vi "Stepper Mover.vi"() -> ()   [LabVIEW 2020]
doc: "Use this template to build a producer/consumer design pattern with events to produce queue items. Use this design pattern instead of the User Interface Event Handler pattern for user interfaces when you want to execute code asynchronously in response to an event without slowing the user interface responsiveness."
panel:
  out "Timeout error":bool
  out "error out":errorcluster
  in  "Velocity":i32
  in  "Init":bool
  in  "Set to Zero":bool
  in  "Stop Motor":bool
  out "Moving":bool
  out "Current Top Position":dbl format="%.1f"
  out "Current Bottom Position":dbl format="%.4f"
  in  "Instrument Address":refnum<visa-resource-name>
  in  "Rotator":T1(ring)=enum."System B 50 mm Magnet"
  in  "Move to Bottom Position (deg or in)":dbl format="%.4f"
  in  "Move to  Top Position (deg)":dbl format="%.1f"
  in  "stop":bool
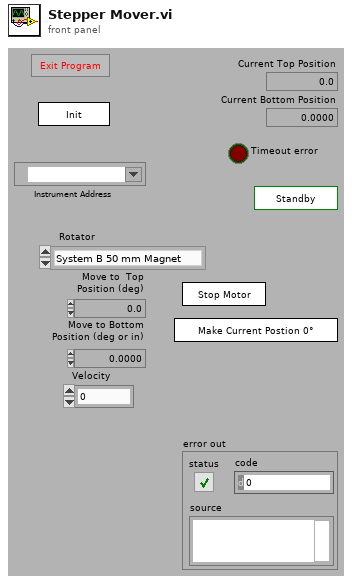
[diagram p1: front panel]
types:
  T1 = enum16{"Dilution Fridge SCM 1", "System A SCM 2", "System B 50 mm Magnet", "He-3 32 mm Magnet", "Portable Dil Fridge Rotator", "Linear Position", "System E Probe 1"}
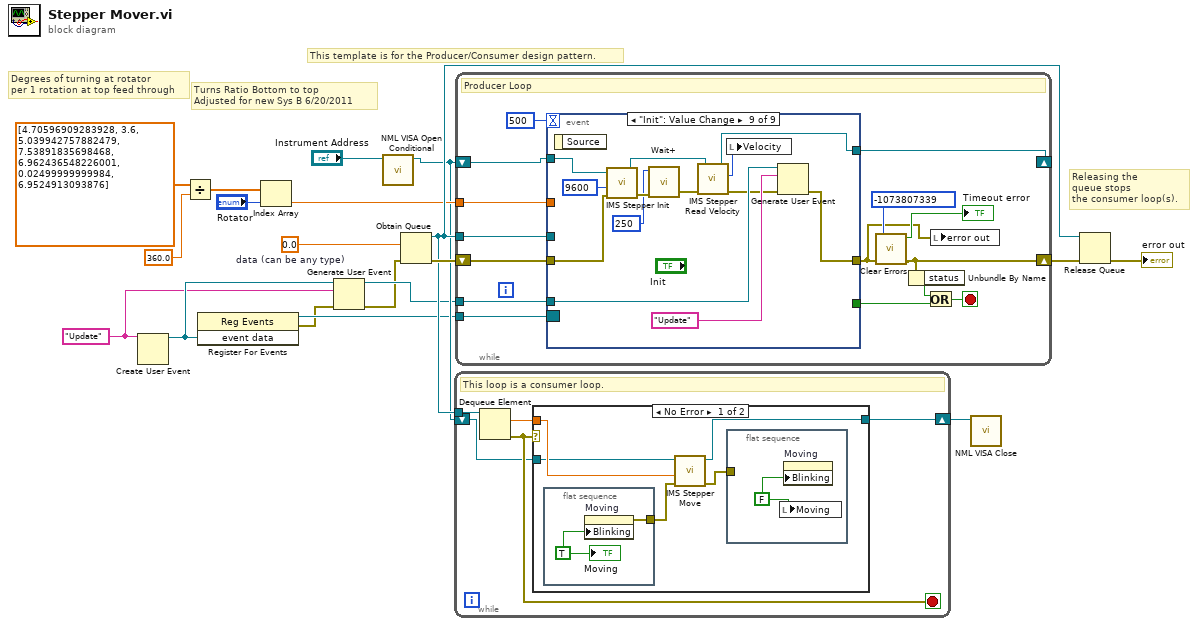
[diagram p0: block diagram]
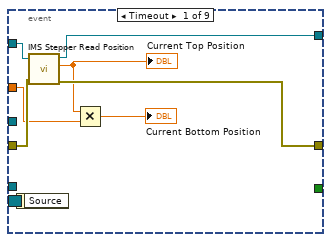
[diagram p3: hidden frame]
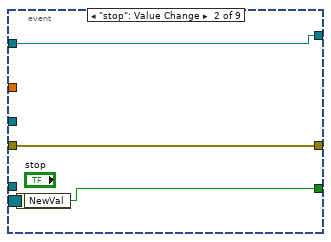
[diagram p4: hidden frame]
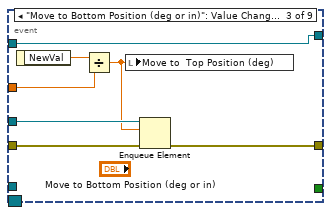
[diagram p5: hidden frame]
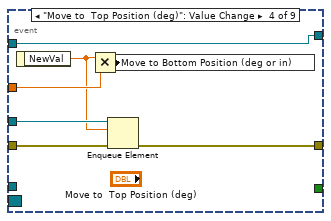
[diagram p6: hidden frame]
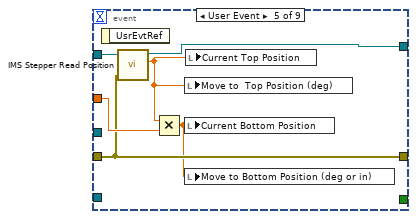
[diagram p7: hidden frame]
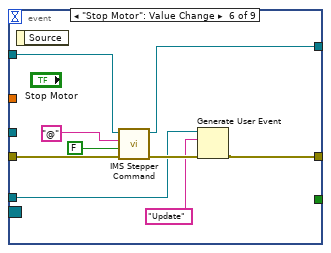
[diagram p8: hidden frame]
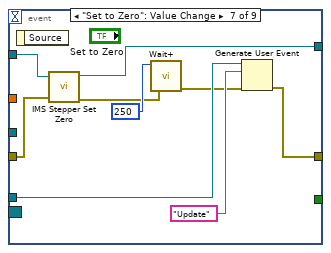
[diagram p9: hidden frame]
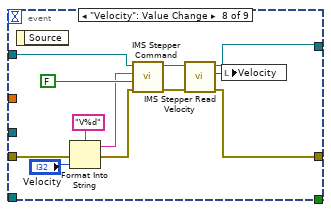
[diagram p10: hidden frame]
diagram:
  w6 = "Update" ("event data")
  w17 = 0.0  # data (can be any type)
  # "Degrees of turning at rotator\nper 1 rotation at top feed through"
  # "Turns Ratio Bottom to top\nAdjusted for new Sys B 6/20/2011"
  # "Releasing the\nqueue stops\nthe consumer loop(s)."
  # "This template is for the Producer/Consumer design pattern."
  n1 = Create User Event(user event datatype=w6) -> (user event=w9:refnum<user-event>)  [unwired: 1 in, 1 out]
  n2 = Divide(x=dbl[] [4.70596909283928, 3.6, 5.039942757882479, 7.53891835698468, 6.962436548226001, 0.02499999999984, 6.9524913093876] ("array"), y=360.0) -> (x/y=w2:dbl[])
  n3 = register-events(w9) -> (reference out=w11:refnum<event-registration>, error out=w10:errorcluster)  [unwired: 2 in]
  n4 = Index Array(array=w2, index="Rotator") -> (element=w13:dbl)
  n5 = Generate User Event(user event=w9, event data cluster=w6, error in=w10) -> (user event out=w8:refnum<user-event>, error out=w7:errorcluster)  [unwired: 1 in]
  n6 = call "NML VISA Open Conditional.vi"("VISA resource name"="Instrument Address") -> ("dup VISA Session"=w12:refnum<visa-resource-name>)  [unwired: 8 in, 2 out]
  n7 = Obtain Queue(element data type=w17, error in (no error)=w7) -> (queue out=w16:refnum<queue>, error out=w19:errorcluster)  [unwired: 3 in, 1 out]
  n8 = while {
    tunnel: w16 -> [w24]
    shift-right: [w20] -> w1
    shift-left: w12 -> [w21]
    stop <- w23 stop-if-true
    # "This loop is a consumer loop."
    n9 = Dequeue Element(queue=w24) -> (element=w22:dbl, error out=w23:errorcluster)  [unwired: 2 in, 2 out]
    n10 = case shown="No Error" w23 {
      tunnel: w22 -> [w29 _]
      tunnel: w21 -> [w28 w33]
      tunnel: [w25 w33] -> w20
      frame No Error {
        n11 = flat-sequence {
          tunnel: [w30] -> w27
          frame #0 {
            w31 = TRUE ("Moving")
            n12 = property on="Moving" class="Bool (strict)"("Blinking"=w31) -> (error out=w30:errorcluster)  [unwired: 2 in, 1 out]
            "Moving" <- w31
          }
        }
        n13 = call "IMS Stepper Move.vi"("error in (no error)"=w27, "Distance"=w29, "Instrument Address"=w28) -> ("error out"=w26:errorcluster, "Instrument Address Out"=w25:refnum<visa-resource-name>)  [unwired: 4 in]
        n14 = flat-sequence {
          tunnel: w26 -> [_]
          frame #0 {
            w32 = FALSE ("Moving")
            n15 = local write "Moving"(w32) -> ()
            n16 = property on="Moving" class="Bool (strict)"("Blinking"=w32) -> ()  [unwired: 2 in, 2 out]
          }
        }
      }
      frame Error {
      }
    }
  }
  n17 = while {
    shift-right: [w36] -> w18
    shift-left: w19 -> [w47]
    tunnel: w16 -> [w48]
    tunnel: w13 -> [w41]
    tunnel: w11 -> [w40]
    tunnel: w8 -> [w39]
    shift-right: [w34] -> _
    shift-left: w12 -> [w42]
    stop <- w45 stop-if-true
    # "Producer Loop"
    n18 = event shown="[8] \"Init\": Value Change" {
      selector: w40 -> [_ _ _ _ _ _ _ _ _]
      dyn-events: _ -> [_ _ _ _ _ _ _ _ _]
      timeout: 500 -> [_ _ _ _ _ _ _ _ _]
      tunnel: w48 -> [_ _ w65 w72 _ _ _ _ _]
      tunnel: w47 -> [w55 w58 w64 w71 w76 w85 w96 w104 w118]
      tunnel: [w52 w58 w63 w70 w76 w83 w94 w99 w121] -> w35
      tunnel: [_ w57 _ _ _ _ _ _ _] -> w46
      tunnel: w42 -> [w54 w56 w59 w66 w77 w87 w95 w101 w110]
      tunnel: w41 -> [w53 _ w62 w69 w78 _ _ _ _]
      tunnel: w39 -> [_ _ _ _ _ w81 w93 _ w120]
      tunnel: [w49 w56 w59 w66 w73 w79 w88 w98 w111] -> w34
      event Timeout {
        n19 = event-data() -> ()  [unwired: 1 in, 1 out]
        n20 = call "IMS Stepper Read Position.vi"("Instrument Address"=w54, "error in (no error)"=w55) -> ("Instrument Address Out"=w49:refnum<visa-resource-name>, "Response"=w51:dbl, "error out"=w52:errorcluster)  [unwired: 2 in]
        "Current Top Position" <- w51
        n21 = Multiply(x=w51, y=w53) -> (x*y=→"Current Bottom Position":dbl)
      }
      event "stop": Value Change {
        n22 = event-data() -> ("NewVal"=w57:bool)  [unwired: 1 in]
      }
      event "Move to Bottom Position (deg or in)": Value Change {
        n23 = event-data() -> ("NewVal"=w61:dbl)  [unwired: 1 in]
        n24 = Divide(x=w61, y=w62) -> (x/y=w60:dbl)
        n25 = local write "Move to  Top Position (deg)"(w60) -> ()
        n26 = Enqueue Element(queue=w65, element=w60, error in (no error)=w64) -> (error out=w63:errorcluster)  [unwired: 1 in, 2 out]
      }
      event "Move to  Top Position (deg)": Value Change {
        n27 = event-data() -> ("NewVal"=w68:dbl)  [unwired: 1 in]
        n28 = Multiply(x=w68, y=w69) -> (x*y=w67:dbl)
        n29 = local write "Move to Bottom Position (deg or in)"(w67) -> ()
        n30 = Enqueue Element(queue=w72, element=w68, error in (no error)=w71) -> (error out=w70:errorcluster)  [unwired: 1 in, 2 out]
      }
      event User Event {
        n31 = event-data() -> ()  [unwired: 1 in, 1 out]
        n32 = call "IMS Stepper Read Position.vi"("Instrument Address"=w77, "error in (no error)"=w76) -> ("Instrument Address Out"=w73:refnum<visa-resource-name>, "Response"=w75:dbl)  [unwired: 2 in, 1 out]
        n33 = Multiply(x=w75, y=w78) -> (x*y=w74:dbl)
        n34 = local write "Move to  Top Position (deg)"(w75) -> ()
        n35 = local write "Current Bottom Position"(w74) -> ()
        n36 = local write "Move to Bottom Position (deg or in)"(w74) -> ()
        n37 = local write "Current Top Position"(w75) -> ()
      }
      event "Stop Motor": Value Change {
        n38 = event-data() -> ()  [unwired: 1 in, 1 out]
        n39 = call "IMS Stepper Command.vi"("error in (no error)"=w85, "Mode"=FALSE, "Command"="@", "Instrument Address"=w87) -> ("error out"=w82:errorcluster, "Instrument Address Out"=w79:refnum<visa-resource-name>)  [unwired: 2 in, 2 out]
        n40 = Generate User Event(user event=w81, event data cluster="Update" ("event data"), error in=w82) -> (error out=w83:errorcluster)  [unwired: 1 in, 1 out]
      }
      event "Set to Zero": Value Change {
        n41 = event-data() -> ()  [unwired: 1 in, 1 out]
        n42 = call "IMS Stepper Set Zero.vi"("Instrument Address"=w95, "error in (no error)"=w96) -> ("Instrument Address Out"=w88:refnum<visa-resource-name>, "error out"=w90:errorcluster)  [unwired: 3 in]
        n43 = call "Wait+.vi"("Error In"=w90, "milliseconds to wait"=u32 250) -> ("Error Out"=w89:errorcluster)  [unwired: 4 in, 1 out]
        n44 = Generate User Event(user event=w93, event data cluster="Update" ("event data"), error in=w89) -> (error out=w94:errorcluster)  [unwired: 1 in, 1 out]
      }
      event "Velocity": Value Change {
        n45 = event-data() -> ()  [unwired: 1 in, 1 out]
        n46 = Format Into String(format string="V%d", error in=w104, "Velocity") -> (resulting string=w105:string, error out=w103:errorcluster)  [unwired: 1 in]
        n47 = call "IMS Stepper Command.vi"("error in (no error)"=w103, "Mode"=FALSE, "Command"=w105, "Instrument Address"=w101) -> ("error out"=w102:errorcluster, "Instrument Address Out"=w97:refnum<visa-resource-name>)  [unwired: 2 in, 2 out]
        n48 = call "IMS Stepper Read Velocity.vi"("error in (no error)"=w102, "Instrument Address"=w97) -> ("error out"=w99:errorcluster, "Velocity"=w100:i32, "dup VISA Resource Name"=w98:refnum<visa-resource-name>)  [unwired: 3 in]
        n49 = local write "Velocity"(w100) -> ()
      }
      event "Init": Value Change {
        n50 = event-data() -> ()  [unwired: 1 in, 1 out]
        n51 = call "IMS Stepper Init.vi"("error in (no error)"=w118, "Baud Rate"=u32 9600, "Instrument Address"=w110) -> ("error out"=w113:errorcluster, "dup VISA Resource Name"=w109:refnum<visa-resource-name>)  [unwired: 2 in, 1 out]
        n52 = call "Wait+.vi"("Error In"=w113, "milliseconds to wait"=u32 250) -> ("Error Out"=w114:errorcluster)  [unwired: 4 in, 1 out]
        n53 = call "IMS Stepper Read Velocity.vi"("error in (no error)"=w114, "Instrument Address"=w109) -> ("error out"=w116:errorcluster, "Velocity"=w115:i32, "dup VISA Resource Name"=w111:refnum<visa-resource-name>)  [unwired: 3 in]
        n54 = local write "Velocity"(w115) -> ()
        n55 = Generate User Event(user event=w120, event data cluster="Update" ("event data"), error in=w116) -> (error out=w121:errorcluster)  [unwired: 1 in, 1 out]
      }
    }
    n56 = call <vilib>:"Clear Errors.vi"("error in (no error)"=w35, "specific error code to clear (0: all)"=-1073807339) -> ("error out"=w36:errorcluster, "specific error cleared?"=→"Timeout error":bool)  [unwired: 4 in]
    n57 = Unbundle By Name(w36) -> ("status"=w44:bool)
    n58 = Or(x=w44, y=w46) -> (x .or. y?=w45:bool)
    n59 = local write "error out"(w35) -> ()
  }
  n60 = call "NML VISA Close.vi"("VISA resource name"=w1) -> ()  [unwired: 10 in, 1 out]
  n61 = Release Queue(queue=w16, error in (no error)=w18) -> (error out=→"error out":errorcluster)  [unwired: 1 in, 2 out]
